vi "InchesToArmUnits.vi"(11 "Inches":dbl) -> (3 "Sensor Units":i32)   [LabVIEW 2018]
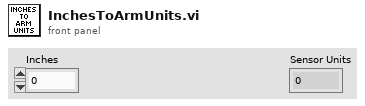
[diagram p1: front panel]
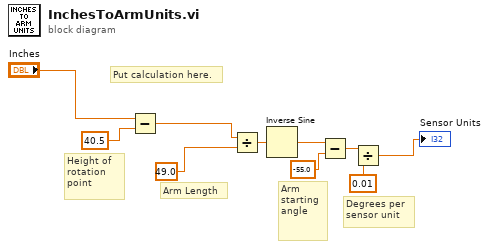
[diagram p0: block diagram]
diagram:
  # "Degrees per sensor unit"
  # "Arm starting angle"
  # "Arm Length"
  # "Height of rotation point"
  # "Put calculation here."
  n1 = Subtract(x="Inches", y=40.5) -> (x-y=w8:dbl)
  n2 = Divide(x=w8, y=49.0 ("Inches")) -> (x/y=w6:dbl)
  n3 = Inverse Sine(1:w6) -> (0:w5:dbl)
  n4 = Subtract(x=w5, y=-55.0) -> (x-y=w3:dbl)
  n5 = Divide(x=w3, y=0.01) -> (x/y=→"Sensor Units":dbl)
